vi "sv_Enumeration (Function Type).vi"() -> (2 "function type strings":T2, 3 "function type values":T1[](array[typedef]))   [LabVIEW 2017, in "SoundVib_UFF58.lvlib"]
uses:
  <vilib>/addons/Sound and Vibration/svt_UFF58/SoundVib_UFF58.lvlib
  <vilib>/addons/Sound and Vibration/svt_UFF58/subVIs/sv_FunctionType Array.ctl
  <vilib>/addons/Sound and Vibration/svt_UFF58/subVIs/sv_FunctionType.ctl
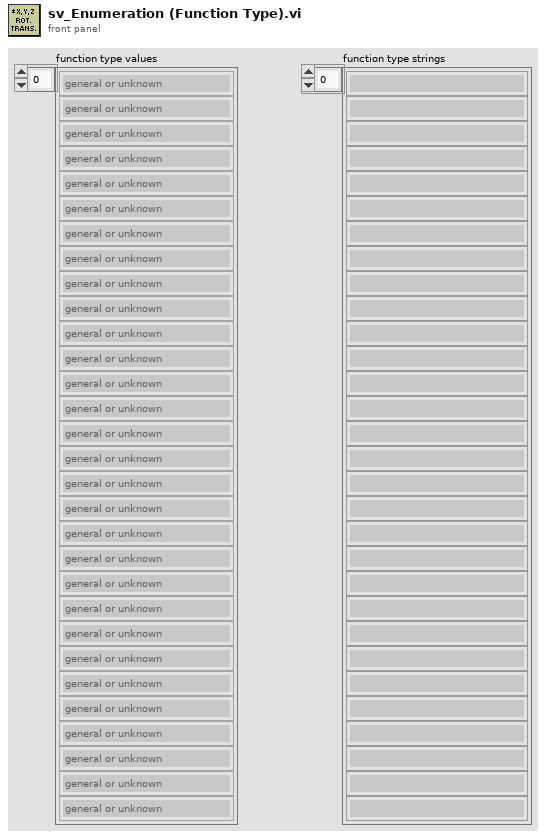
[diagram p1: front panel]
types:
  T1 = typedef "SoundVib_UFF58.lvlib/sv_FunctionType.ctl" = enum16{"general or unknown", "time response", "auto spectrum", "cross spectrum", "frequency response function", "transmissibility", "coherence", "auto correlation", "cross correlation", "power spectral density (PSD)", "energy spectral density (ESD)", "probability density function", "spectrum", "cumulative frequency distribution", "peaks valley", "stress/cycles", "strain/cycles", "orbit", "mode indicator function", "force pattern", "partial power", "partial coherence", "eigenvalue", "eigenvector", "shock response spectrum", "finite impulse response filter", "multiple coherence", "order function", "phase compensation"}
  T2 = typedef "SoundVib_UFF58.lvlib/sv_FunctionType Array.ctl" = string[]
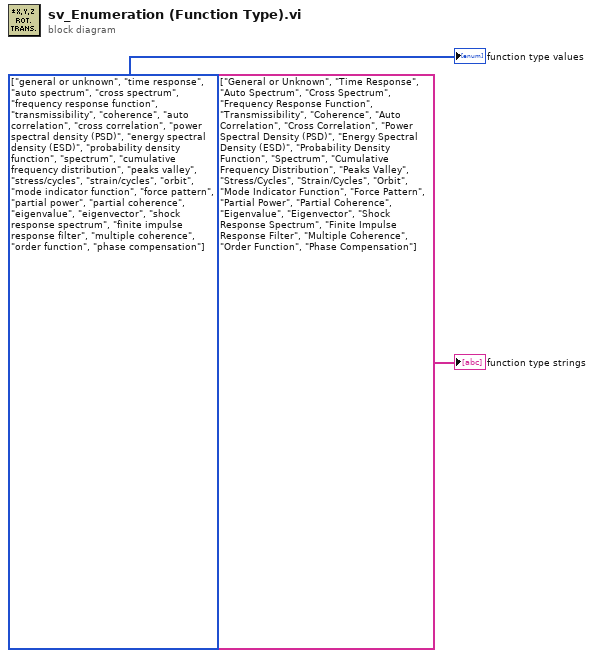
[diagram p0: block diagram]
diagram:
  w2 = T1[] [enum."general or unknown", enum."time response", enum."auto spectrum", enum."cross spectrum", enum."frequency response function", enum."transmissibility", enum."coherence", enum."auto correlation", enum."cross correlation", enum."power spectral density (PSD)", enum."energy spectral density (ESD)", enum."probability density function", enum."spectrum", enum."cumulative frequency distribution", enum."peaks valley", enum."stress/cycles", enum."strain/cycles", enum."orbit", enum."mode indicator function", enum."force pattern", enum."partial power", enum."partial coherence", enum."eigenvalue", enum."eigenvector", enum."shock response spectrum", enum."finite impulse response filter", enum."multiple coherence", enum."order function", enum."phase compensation"] items=["general or unknown", "time response", "auto spectrum", "cross spectrum", "frequency response function", "transmissibility", "coherence", "auto correlation", "cross correlation", "power spectral density (PSD)", "energy spectral density (ESD)", "probability density function", "spectrum", "cumulative frequency distribution", "peaks valley", "stress/cycles", "strain/cycles", "orbit", "mode indicator function", "force pattern", "partial power", "partial coherence", "eigenvalue", "eigenvector", "shock response spectrum", "finite impulse response filter", "multiple coherence", "order function", "phase compensation"]
  "function type strings" <- T2 ["General or Unknown", "Time Response", "Auto Spectrum", "Cross Spectrum", "Frequency Response Function", "Transmissibility", "Coherence", "Auto Correlation", "Cross Correlation", "Power Spectral Density (PSD)", "Energy Spectral Density (ESD)", "Probability Density Function", "Spectrum", "Cumulative Frequency Distribution", "Peaks Valley", "Stress/Cycles", "Strain/Cycles", "Orbit", "Mode Indicator Function", "Force Pattern", "Partial Power", "Partial Coherence", "Eigenvalue", "Eigenvector", "Shock Response Spectrum", "Finite Impulse Response Filter", "Multiple Coherence", "Order Function", "Phase Compensation"] ("FunctionType")
  "function type values" <- w2
